vi "Read Rotator Position.vi"(8 "error in (no error)":errorcluster) -> (0 "error out":errorcluster)   [LabVIEW 2016]
uses:
  PPMS Global.vi
panel:
  out "Position (Degree)":dbl
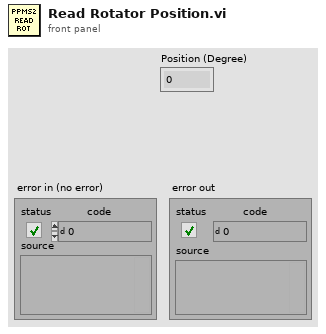
[diagram p1: front panel]
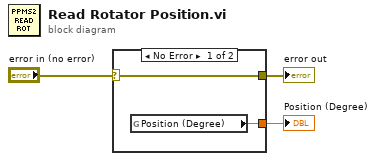
[diagram p0: block diagram]
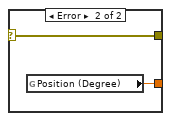
[diagram p2: hidden frame]
diagram:
  n1 = case shown="No Error" "error in (no error)" {
    selector: "error in (no error)" -> [w5 w7]
    tunnel: [w5 w7] -> w2
    tunnel: [w4 w6] -> w1
    frame No Error {
      n2 = global read "PPMS Global.vi" "Position (Degree)"() -> (w4:dbl)
    }
    frame Error {
      n3 = global read "PPMS Global.vi" "Position (Degree)"() -> (w6:dbl)
    }
  }
  "error out" <- w2
  "Position (Degree)" <- w1
